vi "Alicat_PCD_stable.vi"() -> ()   [LabVIEW 2023]
panel:
  in  "stop":bool
  out "Measurement Data":T1
  # "Totalizer Timer"
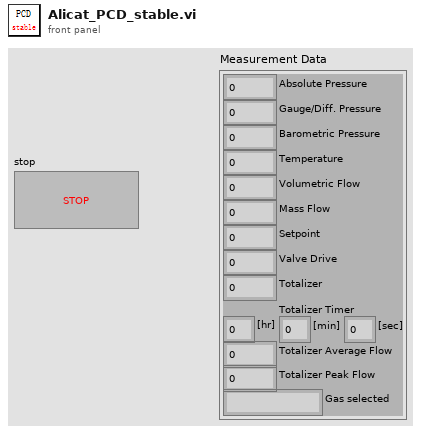
[diagram p1: front panel]
types:
  T1 = cluster{"Absolute Pressure":dbl, "Gauge/Diff. Pressure":dbl, "Barometric Pressure":dbl, "Temperature":dbl, "Volumetric Flow":dbl, "Mass Flow":dbl, "Setpoint":dbl, "Valve Drive":dbl, "Totalizer":dbl, "[hr]":dbl, "[min]":dbl, "[sec]":dbl, "Totalizer Average Flow":dbl, "Totalizer Peak Flow":dbl, "Gas selected":string}
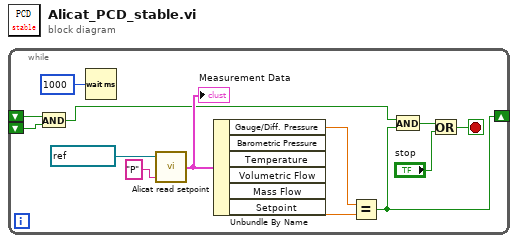
[diagram p0: block diagram]
diagram:
  n1 = while {
    shift-right: [w2] -> _
    shift-left: _ -> [w5]
    shift-left: _ -> [w4]
    stop <- w6 stop-if-true
    n2 = And(x=w5, y=w4) -> (x .and. y?=w3:bool)
    n3 = Wait (ms)(milliseconds to wait=u32 1000) -> ()  [unwired: 1 out]
    n4 = call "Alicat read setpoint.vi"("Unit ID"="P", "ALICAT COM Port"=refnum<visa-resource-name> "COM5") -> ("Measurement Data"=w11:T1)  [unwired: 3 in]
    "Measurement Data" <- w11
    n5 = Unbundle By Name(w11) -> ("Gauge/Diff. Pressure"=w9:dbl, "Setpoint"=w8:dbl)  [unwired: 4 out]
    n6 = Equal?(x=w9, y=w8) -> (x = y?=w2:bool)
    n7 = And(x=w3, y=w2) -> (x .and. y?=w1:bool)
    n8 = Or(x=w1, y="stop") -> (x .or. y?=w6:bool)
  }
